vi "AttackerPenalty2.vi"(4 "AI Parameters":T8={"GotoKick"={"Dist do cone a frente"=150.0, "attacker farback"=1500.0, "Perto"=300.0, "min dist to kick"=150.0, "kick eps"=0.0, "Time to transition"=0.05}, "Attacker"={"CC chute"=0.09, "CC passe"=0.045, "Kick Force"=100.0, "ball-robot Kick"=200.0, "ball-robot Pass"=0.3, "drible\nAttk"=FALSE}, "Defender"={"D max"=1700.0, "Vel p/ robô av"=1000.0, "Kick Force"=100.0, "D atk-def"=0.0, "D farback"=0.0, "drible\ndef"=FALSE, "drible\ngoalie"=FALSE}, "Timeout"={"Field/v in x"=6.0, "Dist Robots"=300, "Dist up in y"=300}, "Pose Striker"={"dist"=200.0, "Numeric"=-4.0, "dist 2"=200.0, "drible\nstriker"=FALSE}, "Dist Stop"=300.0, "D ball out"=200, "D central gap "=150.0, "T pass"=0.0, "Force ++"=0.0, "range kick"=0.0, "Chute alto"=TRUE, "Marcador novo"=TRUE, "drible"=FALSE, "D drible"=300.0, "Versão Striker"=enum."Auto", "Defesa"=enum."ManMark", "Marcador"=enum."Marcar Segundo mais perigoso", "Receptor passe"=enum."Auto", "Área"=enum."Quadrada", "Decisão\nsimples?"=FALSE} {"D drible" format="%#_13g"; "D central gap" format="%#_13g"; "Dist Stop" format="%#_13g"; "Pose Striker"."Numeric" format="%#_13g"; "Defender"."Kick Force" format="%#_13g"; "Defender"."Vel p/ robô av" format="%#_13g"; "Attacker"."ball-robot Kick" format="%#_13g"; "Attacker"."Kick Force" format="%#_13g"; "Attacker"."CC passe" format="%#_13g"; "Attacker"."CC chute" format="%#_13g"; "GotoKick"."kick eps" format="%#_13g"; "GotoKick"."min dist to kick" format="%#_13g"; "GotoKick"."Perto" format="%#_13g"; "GotoKick"."attacker farback" format="%#_13g"; "GotoKick"."Dist do cone a frente" format="%#_13g"}, 7 "IA State Input":T9={"our_robots"=[], "enemy_robots"=[], "balls"=[], "geometry"={"line_width"=0, "field_length"=0, "field_width"=0, "boundary_width"=0, "referee_width"=0, "goal_width"=0, "goal_depth"=0, "goal_wall_width"=0, "center_circle_radius"=0, "defense_radius"=0, "defense_stretch"=0, "free_kick_from_defense_dist"=0, "penalty_spot_from_field_line_dist"=0, "penalty_line_from_spot_dist"=0}, "IA Judge"={"stage"="", "command"="", "our_goalie_id"=0.0, "enemy_goalie_id"=0.0, "command enum"=enum."Halt", "Time"=enum."Azul"}, "Received Timestamp"=timestamp(0 s since 1904-01-01), "Events"={"Touch"=FALSE, "Ball out"=FALSE, "id touch"=0.0, "Ball out of \nVision"=FALSE, "Ball inside \nGoalie area"=FALSE, "Robot not responding"=FALSE, "Robots responding status"=[1.0, 1.0, 1.0, 1.0, 1.0, 1.0], "Enemy Ball \nPossession"=FALSE, "Pass State"=FALSE, "id end of pass"=0.0, "Kick"=FALSE, "Id ini Possession"=0.0, "Ball Possesion"=FALSE, "Id Possesion"=0.0, "Direct Kick"=FALSE, "2nd Strk Ativo"=FALSE}}, 8 "atacando contra?":bool=TRUE, 9 "balls":T6[](array[typedef]), 10 "geometry":T7, 11 "Robot in":T1={"id"=0, "function"=enum."Attacker", "x"=0.0, "y"=0.0, "orientation"=0.0, "v_tangent"=0.0, "v_normal"=0.0, "v_ang"=0.0, "kick_x"=0.0, "kick_z"=0.0, "dribble"=FALSE, "Timestamp"=timestamp(0 s since 1904-01-01), "estimatives"={"est_v_tangent"=0.0, "est_v_normal"=0.0, "est_vx"=0.0, "est_vy"=0.0, "Pos Robot Est"=[]}, "dest_x_kick"=0.0, "dest_y_kick"=0.0, "Gap Coord"=[], "States"=enum."GoToTangent", "Path "=[], "Path  Smooth"=[], "Dest"=[]}) -> (2 "Robot out":T1={"id"=5, "function"=enum."Attacker", "x"=-1842.5054931640625, "y"=520.60986328125, "orientation"=-2.7555055618286133, "v_tangent"=-0.08361641967936218, "v_normal"=-0.20513016702014014, "v_ang"=0.24456003022714357, "kick_x"=0.0, "kick_z"=0.0, "dribble"=FALSE, "Timestamp"=timestamp(2082758857.4639893 s since 1904-01-01), "estimatives"={"est_v_tangent"=0.0, "est_v_normal"=0.0, "est_vx"=0.0, "est_vy"=0.0, "Pos Robot Est"=[]}, "dest_x_kick"=0.0, "dest_y_kick"=0.0, "Gap Coord"=[], "States"=enum."GoToTangent", "Path "=[], "Path  Smooth"=[], "Dest"=[]})   [LabVIEW 2018]
uses:
  Core/AI Input.ctl
  Core/AI Robot.ctl
  Functions Enum.ctl
  AttackerStates.ctl
  Path Planning/RRT/PathDests.ctl
  Path Planning/RRT/PathDest.ctl
  Core/AI Ball.ctl
  Core/Field Size.ctl
  Core/AI Judge.ctl
  Command Enum.ctl
  Util/Events/Events.ctl
  AI Parameters.ctl
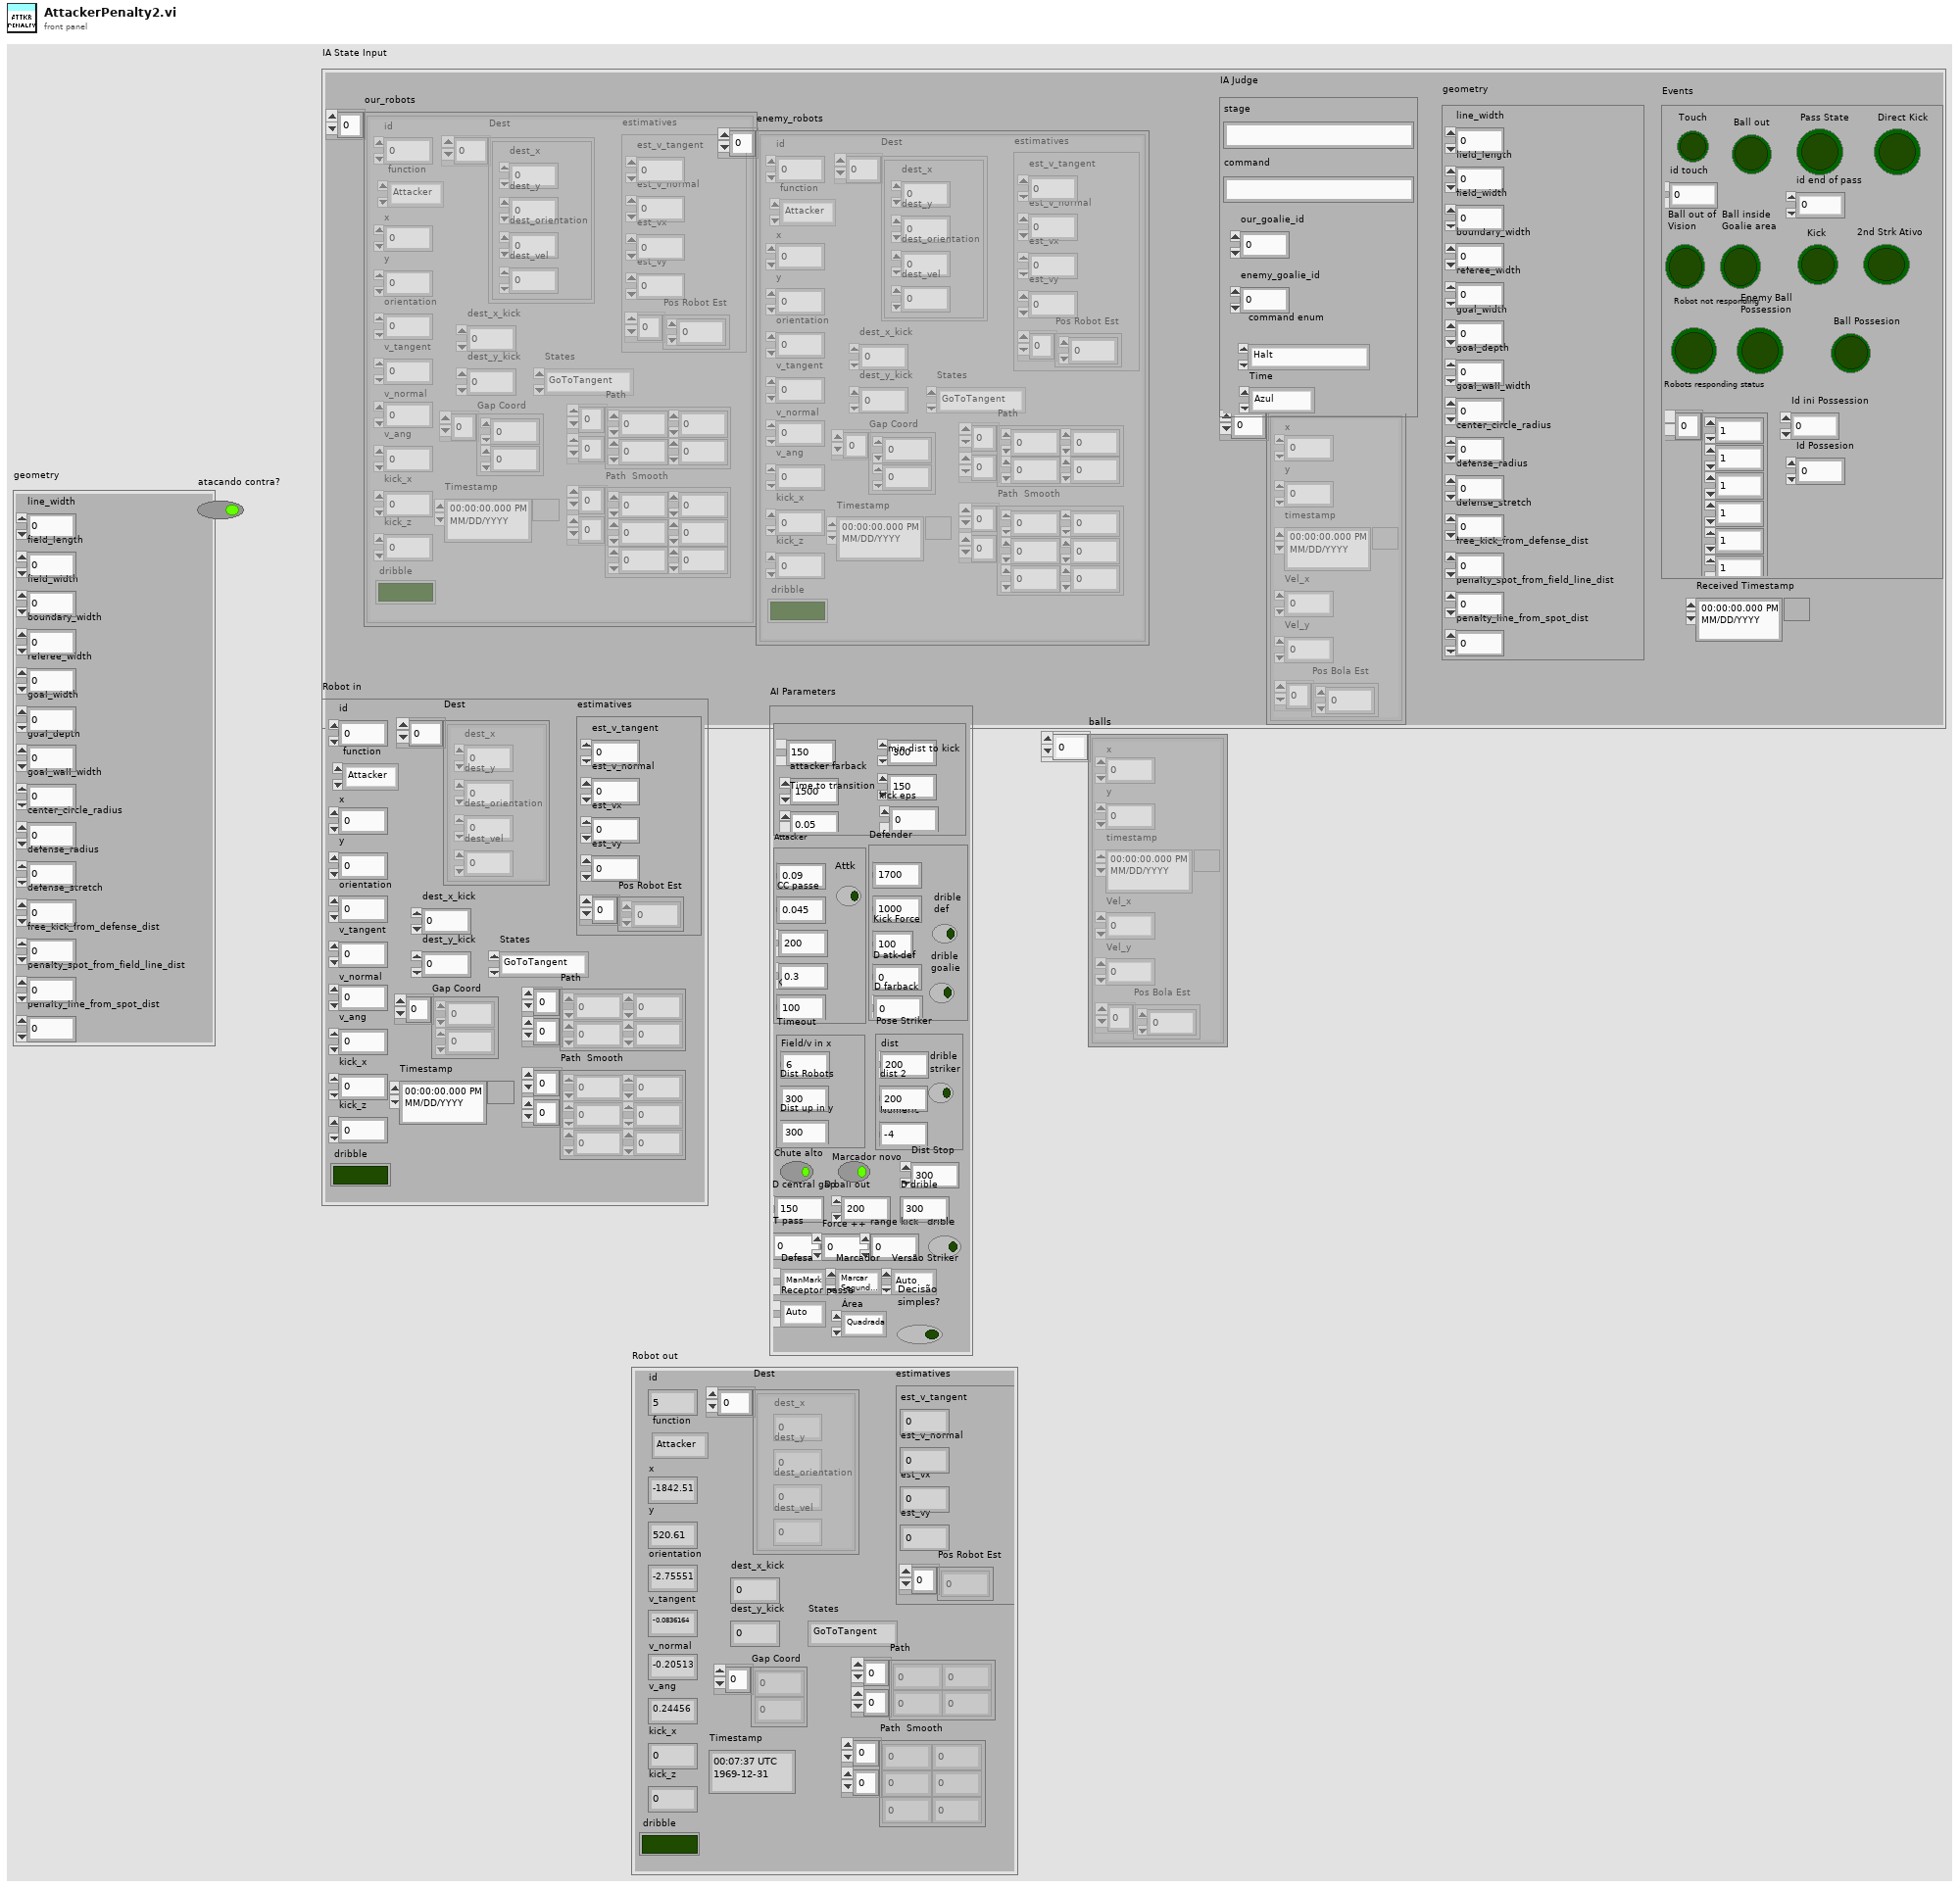
[diagram p1: front panel]
types:
  T1 = typedef "AI Robot.ctl" = cluster{"id":u32, "function":T2, "x":dbl, "y":dbl, "orientation":dbl, "v_tangent":dbl, "v_normal":dbl, "v_ang":dbl, "kick_x":dbl, "kick_z":dbl, "dribble":bool, "Timestamp":timestamp, "estimatives":cluster{"est_v_tangent":dbl, "est_v_normal":dbl, "est_vx":dbl, "est_vy":dbl, "Pos Robot Est":dbl[]}, "dest_x_kick":dbl, "dest_y_kick":dbl, "Gap Coord":dbl[], "States":T3, "Path ":dbl[][], "Path  Smooth":dbl[][], "Dest":T4}
  T2 = typedef "Functions Enum.ctl" = enum16{"2nd Striker", "Attacker", "Goalie", "Defender", "Striker", "Goto 0", "Dummy", "Kicker", "ZigZag 0", "ZigZag 1", "ZigZag 2", "ZigZag 3", "ZigZag 4", "ZigZag 5", "ZigZag 6", "ZigZag 7", "ZigZag 8", ""}
  T3 = typedef "AttackerStates.ctl" = enum16{"Pass", "GoToTangent", "BallGetting", "GoToKick", ""}
  T4 = typedef "PathDests.ctl" = T5[]
  T5 = typedef "PathDest.ctl" = cluster{"dest_x":dbl, "dest_y":dbl, "dest_orientation":dbl, "dest_vel":dbl}
  T6 = typedef "AI Ball.ctl" = cluster{"x":dbl, "y":dbl, "timestamp":timestamp, "Vel_x":dbl, "Vel_y":dbl, "Pos Bola Est":dbl[]}
  T7 = typedef "Field Size.ctl" = cluster{"line_width":u32, "field_length":u32, "field_width":u32, "boundary_width":u32, "referee_width":u32, "goal_width":u32, "goal_depth":u32, "goal_wall_width":u32, "center_circle_radius":u32, "defense_radius":u32, "defense_stretch":u32, "free_kick_from_defense_dist":u32, "penalty_spot_from_field_line_dist":u32, "penalty_line_from_spot_dist":u32}
  T8 = typedef "AI Parameters.ctl" = cluster{"GotoKick":cluster{"Dist do cone a frente":dbl, "attacker farback":dbl, "Perto":dbl, "min dist to kick":dbl, "kick eps":dbl, "Time to transition":dbl}, "Attacker":cluster{"CC chute":dbl, "CC passe":dbl, "Kick Force":dbl, "ball-robot Kick":dbl, "ball-robot Pass":dbl, "drible\nAttk":bool}, "Defender":cluster{"D max":dbl, "Vel p/ robô av":dbl, "Kick Force":dbl, "D atk-def":dbl, "D farback":dbl, "drible\ndef":bool, "drible\ngoalie":bool}, "Timeout":cluster{"Field/v in x":dbl, "Dist Robots":u32, "Dist up in y":u32}, "Pose Striker":cluster{"dist":dbl, "Numeric":dbl, "dist 2":dbl, "drible\nstriker":bool}, "Dist Stop":dbl, "D ball out":i32, "D central gap ":dbl, "T pass":dbl, "Force ++":dbl, "range kick":dbl, "Chute alto":bool, "Marcador novo":bool, "drible":bool, "D drible":dbl, "Versão Striker":enum16{"Auto", "3", "2", "1"}, "Defesa":enum16{"ManMark", "Barreira"}, "Marcador":enum16{"Marcar Segundo mais perigoso", "Marcar o mais perigoso"}, "Receptor passe":enum16{"Auto", "2nd Striker", "Striker"}, "Área":enum16{"Quadrada", "Circular"}, "Decisão\nsimples?":bool}
  T9 = typedef "AI Input.ctl" = cluster{"our_robots":T1[], "enemy_robots":T1[], "balls":T6[], "geometry":T7, "IA Judge":T10, "Received Timestamp":timestamp, "Events":T12}
  T10 = typedef "AI Judge.ctl" = cluster{"stage":string, "command":string, "our_goalie_id":dbl, "enemy_goalie_id":dbl, "command enum":T11, "Time":enum16{"Azul", "Amarelo"}}
  T11 = typedef "Command Enum.ctl" = enum16{"Halt", "Stop", "Force Start", "PKA Normal Start", "Prepare Kickoff Ally", "PKE Normal Start", "Prepare Kickoff Enemy", "Prepare Penalty Ally", "PPA Normal Start", "Prepare Penalty Enemy", "PPE Normal Start", "Direct Free Enemy", "Direct Free Ally", "Indirect Free Enemy", "Indirect Free Ally", "Timeout Enemy", "Timeout Ally", "Goal Enemy", "Goal Ally", "Ball Placement Enemy", "Ball Placement Ally", "Normal Half Time", "Extra Time Break", "Extra Half Time", "None", "Post Game"}
  T12 = typedef "Events.ctl" = cluster{"Touch":bool, "Ball out":bool, "id touch":dbl, "Ball out of \nVision":bool, "Ball inside \nGoalie area":bool, "Robot not responding":bool, "Robots responding status":dbl[], "Enemy Ball \nPossession":bool, "Pass State":bool, "id end of pass":dbl, "Kick":bool, "Id ini Possession":dbl, "Ball Possesion":bool, "Id Possesion":dbl, "Direct Kick":bool, "2nd Strk Ativo":bool}
  T13 = cluster{"CC chute":dbl, "CC passe":dbl, "Kick Force":dbl, "ball-robot Kick":dbl, "ball-robot Pass":dbl, "drible\nAttk":bool}
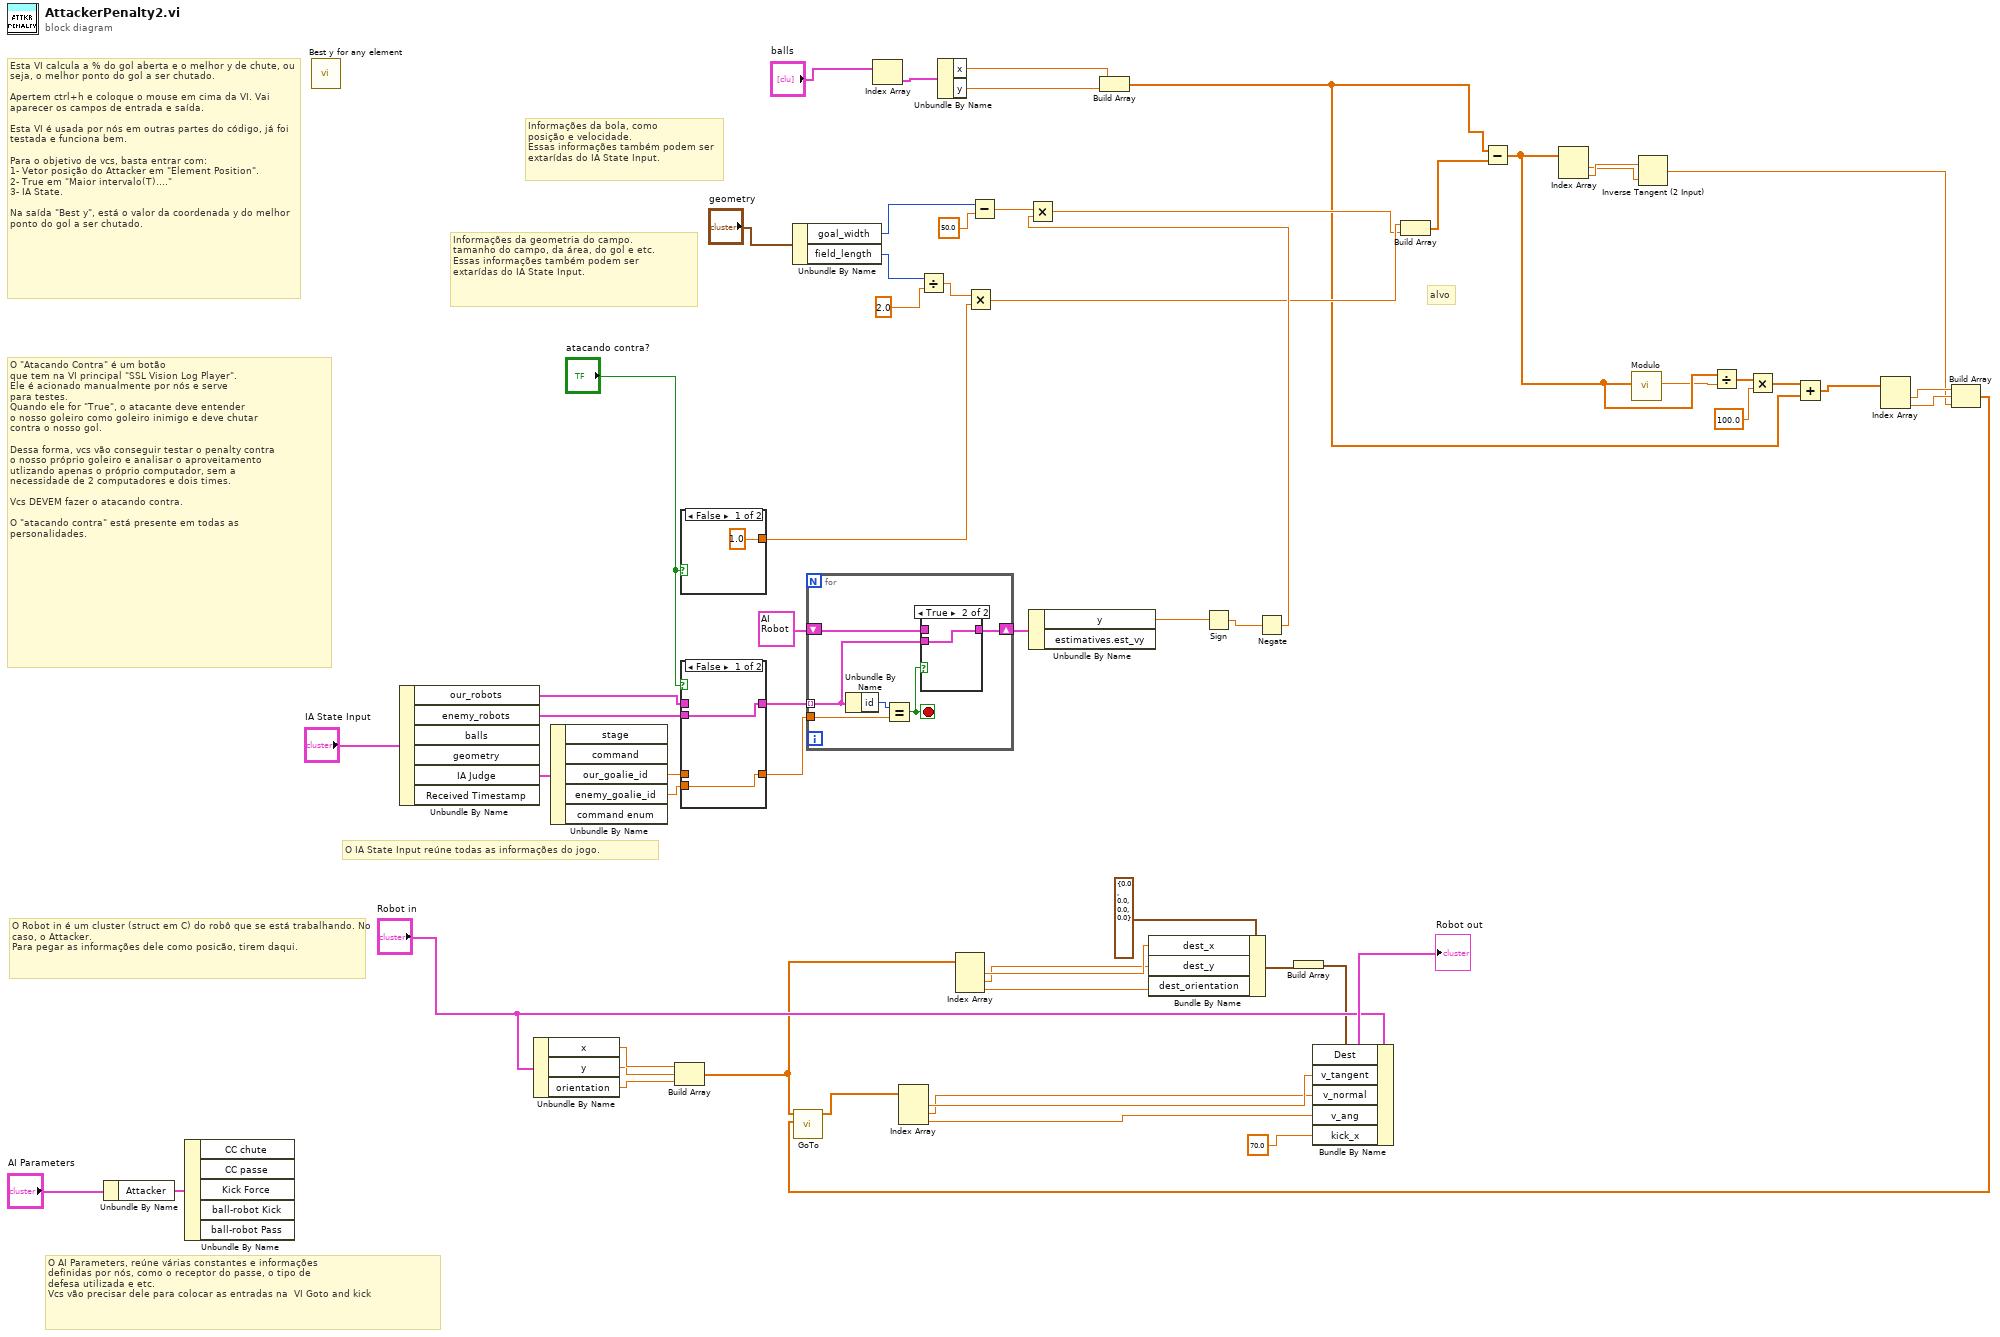
[diagram p0: block diagram]
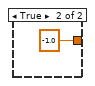
[diagram p3: hidden frame]
diagram:
  # "alvo"
  # "O \"Atacando Contra\" é um botão\nque tem na VI principal \"SSL Vision Log Player\".\nEle é acionado manualmente por nós e serve\npara testes.\nQuando ele for \"True\", o atacante deve entender \no nosso goleiro como goleiro inimigo e deve chutar\ncontra o nosso gol.\n\nDessa forma, vcs vão conseguir testar o penalty contra\no nosso próprio goleiro e analisar o aproveitamento\nutlizando apenas o próprio computador, sem a\nnecessidade de 2 computadores e dois times.\n\nVcs DEVEM fazer o atacando contra. \n\nO \"atacando contra\" está presente em todas as\npersonalidades."
  # "Informações da bola, como\nposição e velocidade.\nEssas informações também podem ser\nextarídas do IA State Input."
  # "Informações da geometria do campo.\ntamanho do campo, da área, do gol e etc.\nEssas informações também podem ser\nextarídas do IA State Input."
  # "O AI Parameters, reúne várias constantes e informações\ndefinidas por nós, como o receptor do passe, o tipo de\ndefesa utilizada e etc.\nVcs vão precisar dele para colocar as entradas na  VI Goto and kick"
  # "O Robot in é um cluster (struct em C) do robô que se está trabalhando. No caso, o Attacker.\nPara pegar as informações dele como posicão, tirem daqui."
  # "O IA State Input reúne todas as informações do jogo."
  # "Esta VI calcula a % do gol aberta e o melhor y de chute, ou seja, o melhor ponto do gol a ser chutado.\n\nApertem ctrl+h e coloque o mouse em cima da VI. Vai aparecer os campos de entrada e saída.\n\nEsta VI é usada por nós em outras partes do código, já foi testada e funciona bem.\n\nPara o objetivo de vcs, basta entrar com:\n1- Vetor posição do Attacker em \"Element Position\".\n2- True em \"Maior intervalo(T)....\"\n3- IA State.\n\nNa saída \"Best y\", está o valor da coordenada y do melhor ponto do gol a ser chutado."
  n1 = Unbundle By Name("AI Parameters") -> ("Attacker"=w61:T13)
  n2 = Unbundle By Name(w61) -> ()  [unwired: 5 out]
  n3 = call "Best y for any element.vi"() -> ()  [unwired: 7 in, 5 out]
  n4 = Unbundle By Name("IA State Input") -> ("our_robots"=w50:T1[], "enemy_robots"=w54:T1[], "IA Judge"=w58:T10)  [unwired: 3 out]
  n5 = Unbundle By Name("Robot in") -> ("x"=w46:dbl, "y"=w45:dbl, "orientation"=w44:dbl)
  n6 = Unbundle By Name(w58) -> ("our_goalie_id"=w51:dbl, "enemy_goalie_id"=w52:dbl)  [unwired: 3 out]
  n7 = Build Array(w46, w45, w44) -> (w14:dbl[])
  n8 = case shown="False" "atacando contra?" {
    tunnel: [1.0 -1.0] -> w29
    frame False {
    }
    frame True {
    }
  }
  n9 = case shown="False" "atacando contra?" {
    tunnel: [w65 w66] -> w55
    tunnel: w54 -> [w65 _]
    tunnel: [w64 w67] -> w53
    tunnel: w52 -> [w64 _]
    tunnel: w51 -> [_ w67]
    tunnel: w50 -> [_ w66]
    frame False {
    }
    frame True {
    }
  }
  n10 = Unbundle By Name("geometry") -> ("goal_width"=w28:u32, "field_length"=w32:u32)
  n11 = for {
    tunnel: w55 -> [w69] mode=indexing
    tunnel: w53 -> [w73]
    shift-right: [w70] -> w49
    shift-left: T1 {"id"=0, "function"=enum."Attacker", "x"=0.0, "y"=0.0, "orientation"=0.0, "v_tangent"=0.0, "v_normal"=0.0, "v_ang"=0.0, "kick_x"=0.0, "kick_z"=0.0, "dribble"=FALSE, "Timestamp"=timestamp(0 s since 1904-01-01), "estimatives"={"est_v_tangent"=0.0, "est_v_normal"=0.0, "est_vx"=0.0, "est_vy"=0.0, "Pos Robot Est"=[]}, "dest_x_kick"=0.0, "dest_y_kick"=0.0, "Gap Coord"=[], "States"=enum."GoToTangent", "Path "=[], "Path  Smooth"=[], "Dest"=[]} ("Robot") -> [w68]
    stop <- w71 stop-if-true
    n12 = Unbundle By Name(w69) -> ("id"=w72:u32)
    n13 = Equal?(x=w72, y=w73) -> (x = y?=w71:bool)
    n14 = case shown="True" w71 {
      tunnel: [w74 w75] -> w70
      tunnel: w69 -> [_ w75]
      tunnel: w68 -> [w74 _]
      frame False {
      }
      frame True {
      }
    }
  }
  n15 = Index Array(array="balls") -> (element=w19:T6)  [unwired: 1 in]
  n16 = Divide(x=w32, y=2.0) -> (x/y=w30:dbl)
  n17 = Unbundle By Name(w19) -> ("x"=w18:dbl, "y"=w17:dbl)
  n18 = Index Array(array=w14) -> (element #1=w38:dbl, element #2=w37:dbl, element #3=w36:dbl)  [unwired: 3 in]
  n19 = Multiply(x=w30, y=w29) -> (x*y=w22:dbl)
  n20 = Subtract(x=w28, y=50.0) -> (x-y=w26:dbl)
  n21 = Unbundle By Name(w49) -> ("y"=w25:dbl)  [unwired: 1 out]
  n22 = Build Array(w18, w17) -> (w2:dbl[])
  n23 = Bundle By Name(cluster=T5 {"dest_x"=0.0, "dest_y"=0.0, "dest_orientation"=0.0, "dest_vel"=0.0} ("Dest"), "dest_x"=w38, "dest_y"=w37, "dest_orientation"=w36) -> (w35:T5)
  n24 = Sign(1:w25) -> (0:w24:dbl)
  n25 = Negate(x=w24) -> (-x=w23:dbl)
  n26 = Multiply(x=w26, y=w23) -> (x*y=w21:dbl)
  n27 = Build Array(w35) -> (w34:T5[])
  n28 = Build Array(w22, w21) -> (w1:dbl[])
  n29 = Subtract(x=w2, y=w1) -> (x-y=w13:dbl[])
  n30 = Index Array(array=w13) -> (element #1=w15:dbl, element #2=w16:dbl)  [unwired: 2 in]
  n31 = call "Modulo.vi"("2D vector"=w13) -> ("Modulo"=w12:dbl)  [unwired: 10 in]
  n32 = Inverse Tangent (2 Input)(1:w15, 2:w16) -> (0:w5:dbl)
  n33 = Divide(x=w13, y=w12) -> (x/y=w11:dbl[])
  n34 = Multiply(x=w11, y=100.0) -> (x*y=w9:dbl[])
  n35 = Add(x=w9, y=w2) -> (x+y=w8:dbl[])
  n36 = Index Array(array=w8) -> (element #1=w7:dbl, element #2=w6:dbl)  [unwired: 2 in]
  n37 = Build Array(w7, w6, w5) -> (w4:dbl[])
  n38 = call "GoTo.vi"("Target"=w4, "Position"=w14) -> ("Output\nVelocity"=w43:dbl[])  [unwired: 8 in, 1 out]
  n39 = Index Array(array=w43) -> (element #1=w42:dbl, element #2=w41:dbl, element #3=w40:dbl)  [unwired: 3 in]
  n40 = Bundle By Name(cluster="Robot in", "Dest"=w34, "v_tangent"=w42, "v_normal"=w41, "v_ang"=w40, "kick_x"=70.0) -> (→"Robot out":T1)
